vi "CorrectTDMSFile.vi"(4 "entrée d'erreur (pas d'erreur)":errorcluster, 7 "chemin du fichier":path) -> (0 "sortie d'erreur":errorcluster)   [LabVIEW 2017]
panel:
  out "TabUnits":string[](array[string])
  out "TabNoms":string[](array[string])
  out "Graphe":waveform(dbl)[](graph)
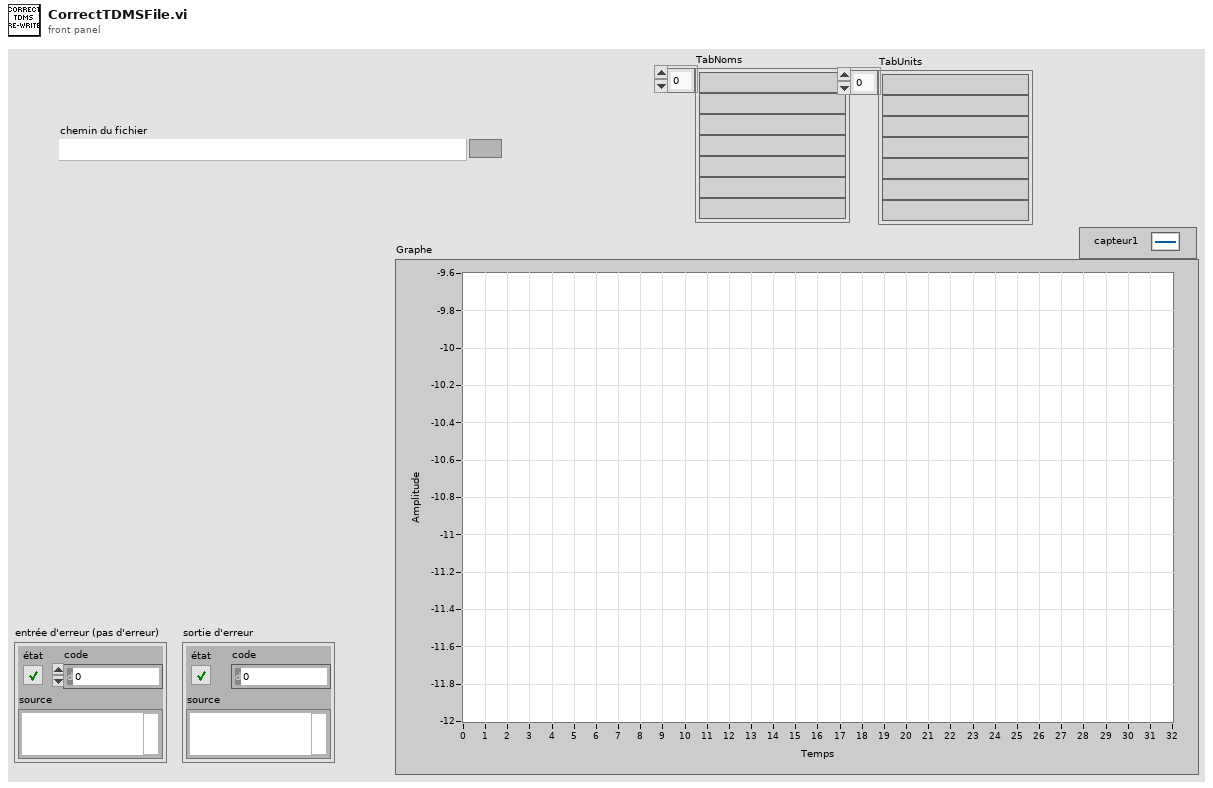
[diagram p1: front panel]
types:
  T1 = enum16{"open", "open or create", "create or replace", "create", "open (read-only)"}
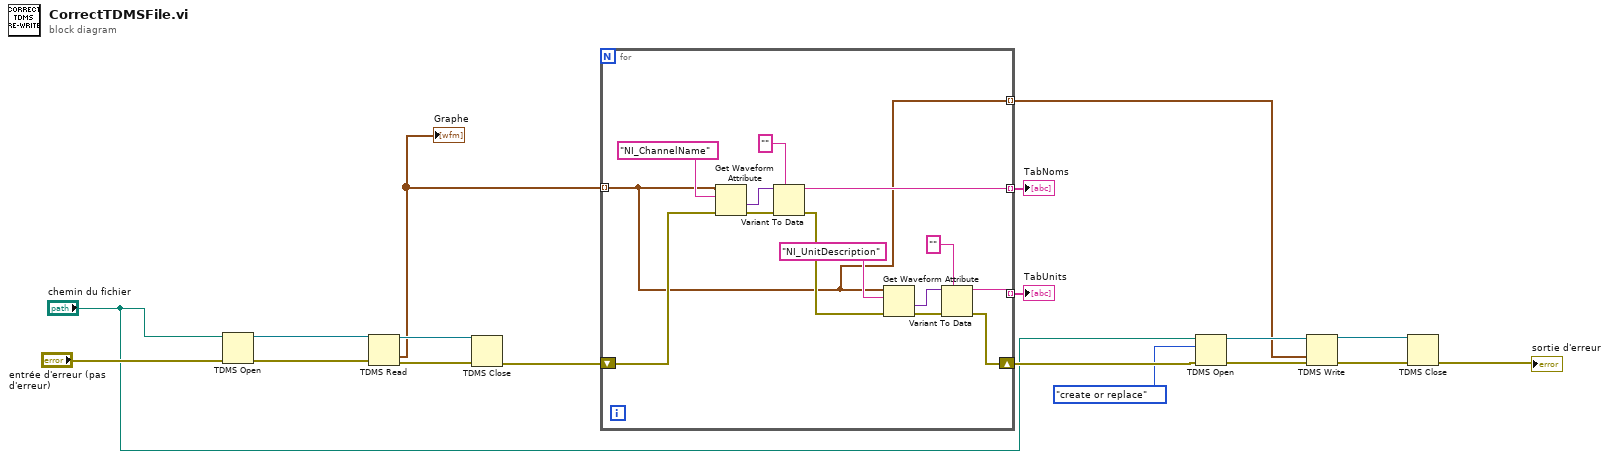
[diagram p0: block diagram]
diagram:
  n1 = TDMS Open(8:"entrée d'erreur (pas d'erreur)", 11:"chemin du fichier") -> (0:w16:errorcluster, 3:w17:refnum<k34>)  [unwired: 5 in]
  n2 = TDMS Read(0:w17, 11:w16) -> (4:w15:refnum<k34>, 10:w13:waveform(dbl)[], 15:w14:errorcluster)  [unwired: 6 in, 3 out]
  "Graphe" <- w13
  n3 = TDMS Close(8:w14, 11:w15) -> (0:w12:errorcluster)  [unwired: 1 out]
  n4 = for {
    tunnel: w13 -> [w19] mode=indexing
    tunnel: [w28] -> w11 mode=indexing
    shift-right: [w20] -> w9
    shift-left: w12 -> [w31]
    tunnel: [w21] -> w10 mode=indexing
    tunnel: [w19] -> w3 mode=indexing
    n5 = Get Waveform Attribute(4:w31, 6:"NI_ChannelName" ("nom"), 7:w19) -> (0:w27:errorcluster, 1:w30:variant)  [unwired: 1 in, 2 out]
    n6 = Variant To Data(error in=w27, type="" ("nom"), Variant=w30) -> (data=w28:string, error out=w22:errorcluster)
    n7 = Get Waveform Attribute(4:w22, 6:"NI_UnitDescription" ("nom"), 7:w19) -> (0:w26:errorcluster, 1:w24:variant)  [unwired: 1 in, 2 out]
    n8 = Variant To Data(error in=w26, type="" ("nom"), Variant=w24) -> (data=w21:string, error out=w20:errorcluster)
  }
  "TabNoms" <- w11
  "TabUnits" <- w10
  n9 = TDMS Open(8:w9, 10:T1."create or replace" ("opération (0 : open)"), 11:"chemin du fichier") -> (0:w8:errorcluster, 3:w4:refnum<k34>)  [unwired: 4 in]
  n10 = TDMS Write(0:w4, 9:w3, 11:w8) -> (4:w2:refnum<k34>, 15:w7:errorcluster)  [unwired: 3 in, 2 out]
  n11 = TDMS Close(8:w7, 11:w2) -> (0:→"sortie d'erreur":errorcluster)  [unwired: 1 out]
